vi "Calculate X Y Waveform Voltage Out Whole Image.vi"(7 "Raster Scan Direction":T1, 8 "Y Flyback":dbl[][](graph), 9 "Y Waveform":dbl[](graph), 10 "X Flyback":dbl[][](graph), 11 "X Waveform":dbl[](graph)) -> (0 "Start Acq Trigger":bool[](array[boolean]), 1 "Y Waveform Out":dbl[](graph), 2 "DO":u32[](graph), 3 "X Waveform Out":dbl[](graph), 4 "Digital Line Acq":bool[](array[boolean]), 5 "XY Waveform Out":dbl[][](graph))   [LabVIEW 2018]
uses:
  Controls/Scan Direction.ctl
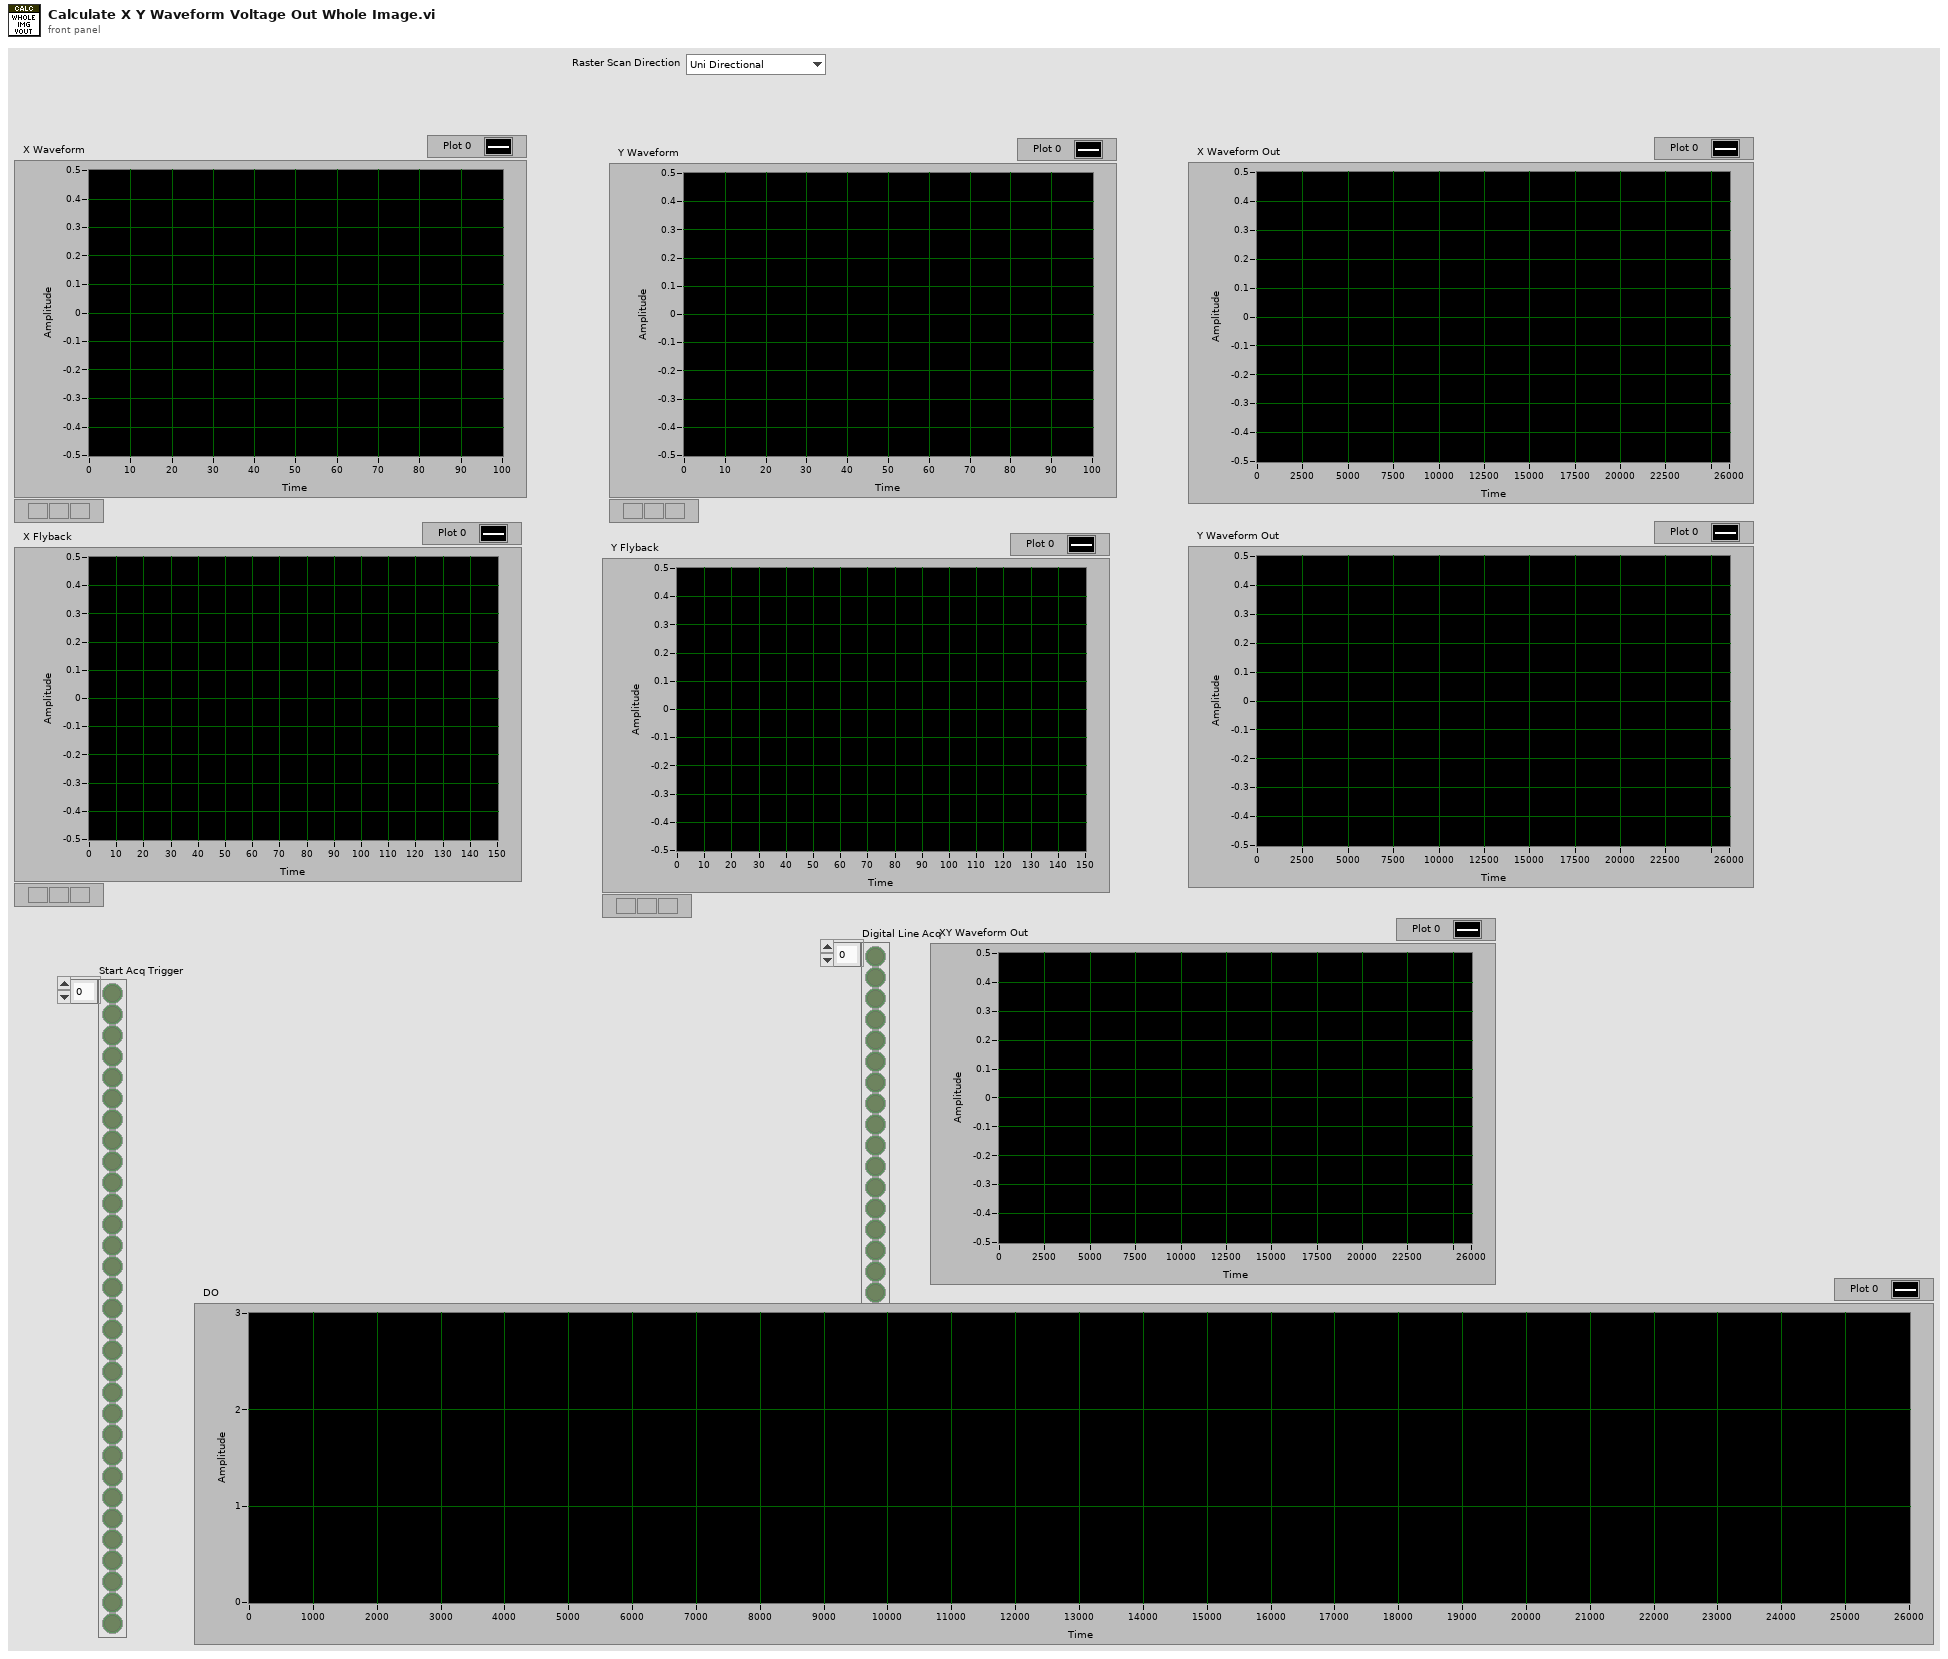
[diagram p1: front panel]
types:
  T1 = typedef "Scan Direction.ctl" = enum16{"Uni Directional", "Bi Directional", "None"}
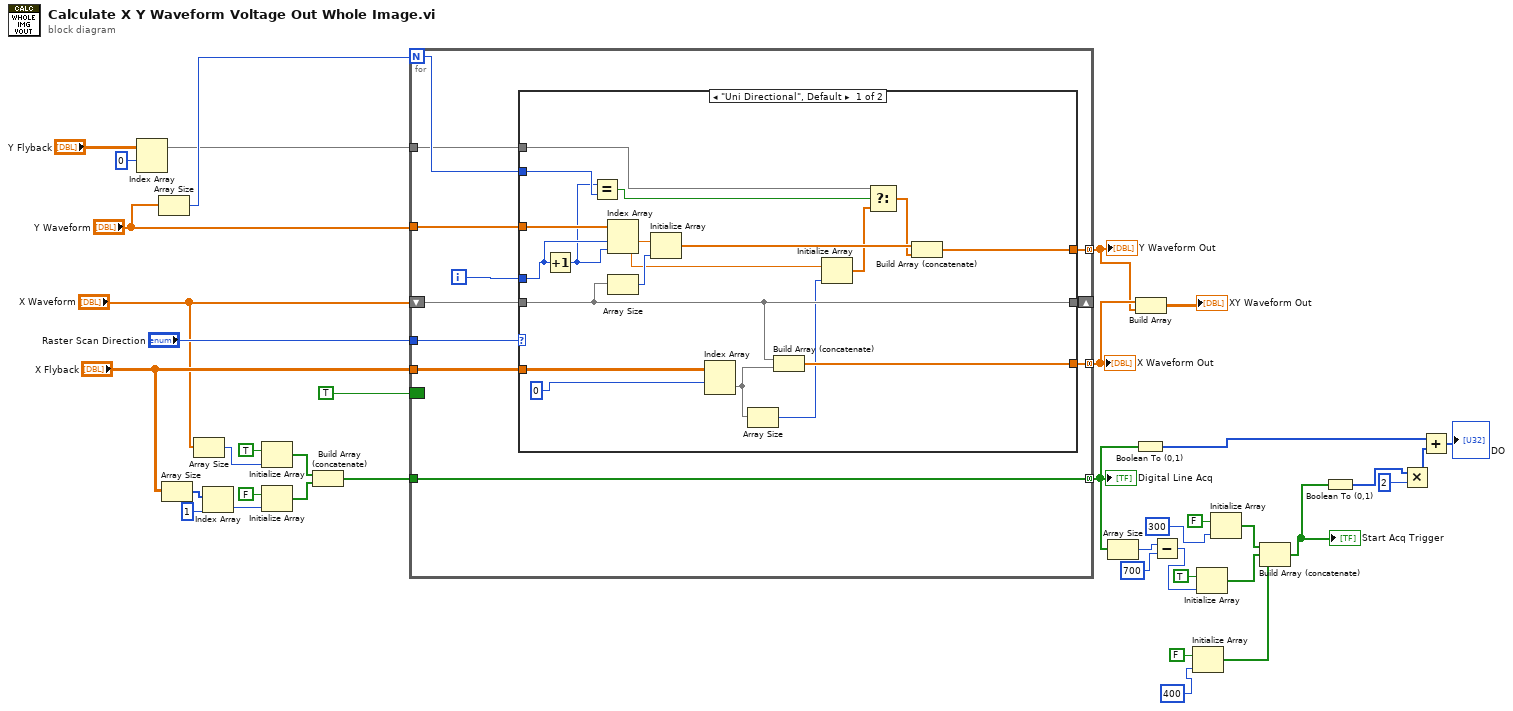
[diagram p0: block diagram]
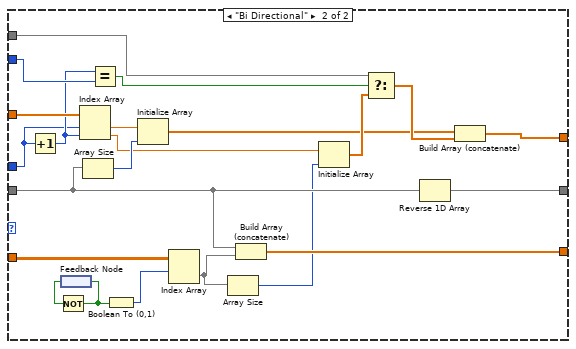
[diagram p2: hidden frame]
diagram:
  n1 = Index Array(array="Y Flyback", index (row)=0) -> (element=w35:dbl[])  [unwired: 1 in]
  n2 = Array Size(array="Y Waveform") -> (size(s)=w37:i32)
  n3 = Array Size(array="X Flyback") -> (size(s)=w28:i32[])
  n4 = Array Size(array="X Waveform") -> (size(s)=w23:i32)
  n5 = Index Array(array=w28, index=1) -> (element=w27:i32)
  n6 = Initialize Array(TRUE, w23) -> (w22:bool[])
  n7 = Initialize Array(FALSE, w27) -> (w21:bool[])
  n8 = Build Array (concatenate)(w22, w21) -> (w18:bool[])
  n9 = for {
    N: w37 -> [w42]
    shift-right: [w50] -> _
    shift-left: "X Waveform" -> [w49]
    tunnel: "Raster Scan Direction" -> [w48]
    tunnel: "Y Waveform" -> [w44]
    tunnel: "X Flyback" -> [w47]
    tunnel: [w45] -> w33 mode=concatenating
    tunnel: [w43] -> w32 mode=concatenating
    tunnel: w35 -> [w41]
    border: TRUE -> [_]
    tunnel: w18 -> [w40]
    tunnel: [w40] -> w5 mode=concatenating
    i -> [w46]
    n10 = case shown="\"Uni Directional\", Default" w48 {
      tunnel: [w63 w91] -> w50
      tunnel: w49 -> [w63 w81]
      tunnel: w47 -> [w69 w90]
      tunnel: w46 -> [w57 w83]
      tunnel: [w67 w89] -> w45
      tunnel: w44 -> [w66 w85]
      tunnel: [w58 w74] -> w43
      tunnel: w42 -> [w56 w86]
      tunnel: w41 -> [w52 w87]
      frame "Uni Directional", Default {
        n11 = Increment(x=w57) -> (x+1=w51:i32)
        n12 = Equal?(x=w51, y=w56) -> (x = y?=w55:bool)
        n13 = Index Array(array=w66, index #1=w57, index #2=w51) -> (element #1=w65:dbl, element #2=w62:dbl)
        n14 = Array Size(array=w63) -> (size(s)=w64:i32)
        n15 = Initialize Array(w65, w64) -> (w59:dbl[])
        n16 = Index Array(array=w69, index (row)=0 ("disabled index (col)")) -> (element=w61:dbl[])  [unwired: 1 in]
        n17 = Array Size(array=w61) -> (size(s)=w60:i32)
        n18 = Build Array (concatenate)(w63, w61) -> (w67:dbl[])
        n19 = Initialize Array(w62, w60) -> (w53:dbl[])
        n20 = Select(t=w52, s=w55, f=w53) -> (s? t:f=w54:dbl[])
        n21 = Build Array (concatenate)(w59, w54) -> (w58:dbl[])
      }
      frame "Bi Directional" {
        n22 = Increment(x=w83) -> (x+1=w84:i32)
        n23 = feedback #1() -> (w72:bool)
        n24 = Not(x=w72) -> (.not. x?=w71:bool)
        n25 = feedback-in #1(w71) -> ()
        n26 = Index Array(array=w85, index #1=w83, index #2=w84) -> (element #1=w82:dbl, element #2=w79:dbl)
        n27 = Array Size(array=w81) -> (size(s)=w80:i32)
        n28 = Equal?(x=w84, y=w86) -> (x = y?=w88:bool)
        n29 = Boolean To (0,1)(Boolean=w71) -> (0, 1=w70:i16)
        n30 = Initialize Array(w82, w80) -> (w73:dbl[])
        n31 = Index Array(array=w90, index (row)=w70) -> (element=w77:dbl[])  [unwired: 1 in]
        n32 = Array Size(array=w77) -> (size(s)=w76:i32)
        n33 = Build Array (concatenate)(w81, w77) -> (w89:dbl[])
        n34 = Initialize Array(w79, w76) -> (w78:dbl[])
        n35 = Select(t=w87, s=w88, f=w78) -> (s? t:f=w75:dbl[])
        n36 = Reverse 1D Array(array=w81) -> (reversed array=w91:dbl[])
        n37 = Build Array (concatenate)(w73, w75) -> (w74:dbl[])
      }
    }
  }
  "X Waveform Out" <- w33
  "Y Waveform Out" <- w32
  "Digital Line Acq" <- w5
  n38 = Array Size(array=w5) -> (size(s)=w17:i32)
  n39 = Boolean To (0,1)(Boolean=w5) -> (0, 1=w3:i16[])
  n40 = Build Array(w33, w32) -> (→"XY Waveform Out":dbl[][])
  n41 = Subtract(x=w17, y=700) -> (x-y=w16:i32)
  n42 = Initialize Array(FALSE, 400 ("dimension size")) -> (w7:bool[])
  n43 = Initialize Array(TRUE, w16) -> (w13:bool[])
  n44 = Initialize Array(FALSE, 300 ("dimension size")) -> (w14:bool[])
  n45 = Build Array (concatenate)(w14, w13, w7) -> (w4:bool[])
  "Start Acq Trigger" <- w4
  n46 = Boolean To (0,1)(Boolean=w4) -> (0, 1=w10:i16[])
  n47 = Multiply(x=w10, y=u32 2) -> (x*y=w12:u32[])
  n48 = Add(x=w3, y=w12) -> (x+y=→"DO":u32[])
